vi "Subvi pixelclock start stop.vi"(0 "Nframes":u8, 1 "Nlines per frame no skips":u16, 2 "Nlines per frame plus skips":u16, 3 "Nlines all":u16, 7 "Lineclock/Pixelclock":T1, 12 "Master trigger":bool, 13 "Linegate timeout":u16) -> (4 "Gated pixelclock change":bool, 6 "Preframegate":bool, 8 "Preframeclock":bool, 10 "Preframe counter":u8, 15 "Frameclock":bool)   [LabVIEW 2017]
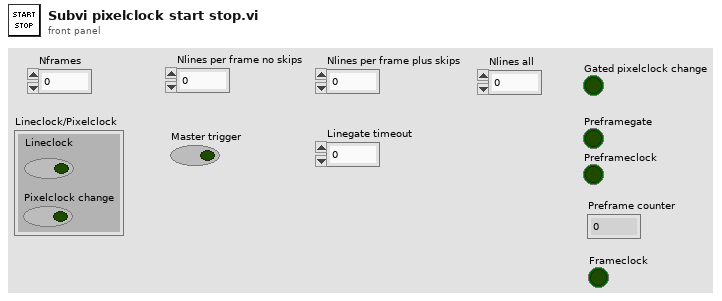
[diagram p1: front panel]
types:
  T1 = cluster{"Pixelclock change":bool, "Lineclock":bool}
  T2 = cluster{cluster{u16, "t":u8}, cluster{bool, u16, u8, bool}, cluster{bool, u16, u8, bool}}
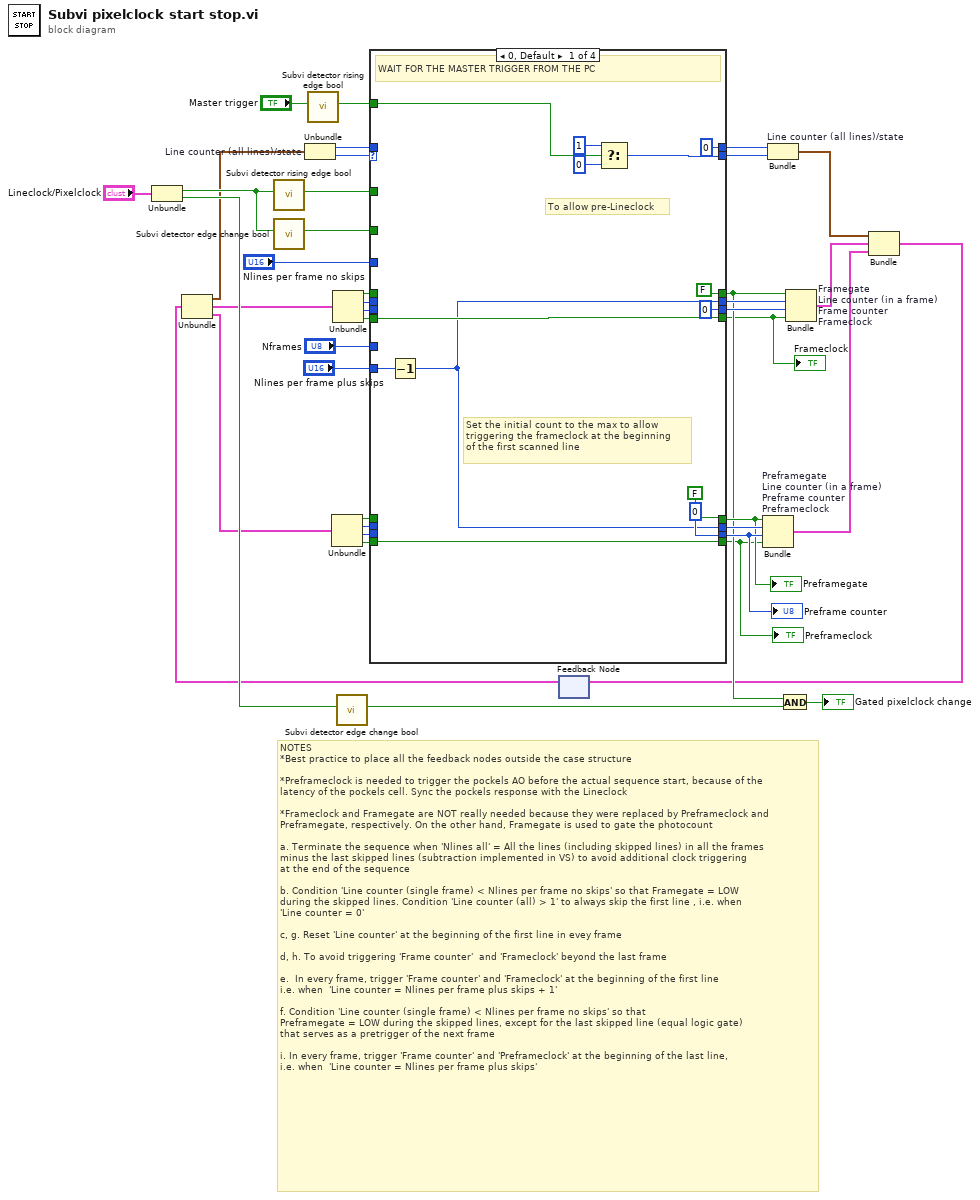
[diagram p0: block diagram]
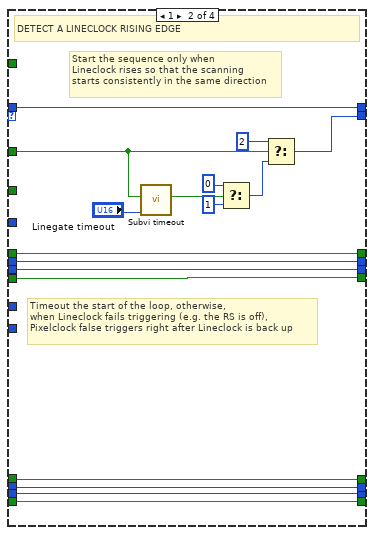
[diagram p2: hidden frame]
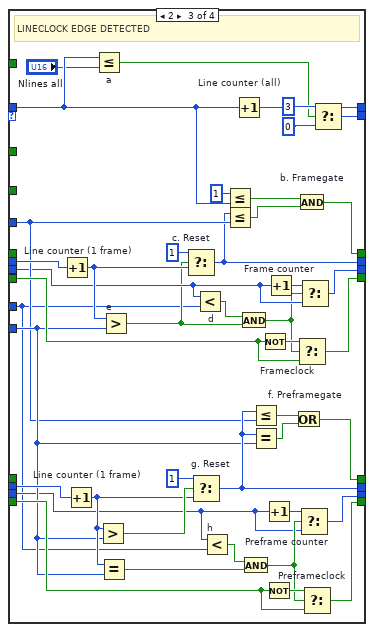
[diagram p3: hidden frame]
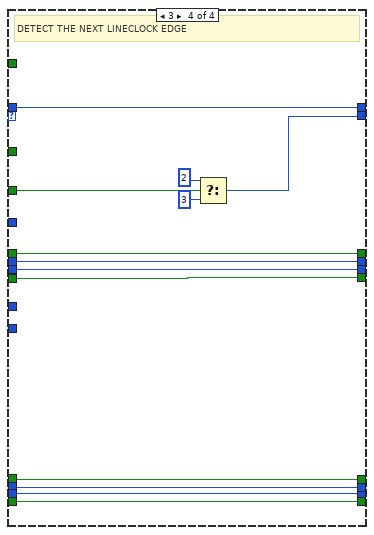
[diagram p4: hidden frame]
diagram:
  # "NOTES\n*Best practice to place all the feedback nodes outside the case structure \n\n*Preframeclock is needed to trigger the pockels AO before the actual sequence start, because of the\nlatency of the pockels cell. Sync the pockels response with the Lineclock\n\n*Frameclock and Framegate are NOT really needed because they were replaced by Preframeclock and \nPreframegate, respectively. On the other hand, Framegate is used to gate the photocount\n\na. Terminate the sequence when 'Nlines all' = All the lines (including skipped lines) in all the frames\nminus the last skipped lines (subtraction implemented in VS) to avoid additional clock triggering\nat the end of the sequence\n\nb. Condition 'Line counter (single frame) < Nlines per frame no skips' so that Framegate = LOW\nduring the skipped lines. Condition 'Line counter (all) > 1' to always skip the first line , i.e. when\n'Line counter = 0'\n\nc, g. Reset 'Line counter' at the beginning of the first line in evey frame\n\nd, h. To avoid triggering 'Frame counter'  and 'Frameclock' beyond the last frame\n\ne.  In every frame, trigger 'Frame counter' and 'Frameclock' at the beginning of the first line\ni.e. when  'Line counter = Nlines per frame plus skips + 1'\n\nf. Condition 'Line counter (single frame) < Nlines per frame no skips' so that\nPreframegate = LOW during the skipped lines, except for the last skipped line (equal logic gate)\nthat serves as a pretrigger of the next frame\n\ni. In every frame, trigger 'Frame counter' and 'Preframeclock' at the beginning of the last line,\ni.e. when  'Line counter = Nlines per frame plus skips'"
  n1 = Unbundle("Lineclock/Pixelclock") -> ("Pixelclock change"=w30:bool, "Lineclock"=w29:bool)
  n2 = call "Subvi detector rising edge bool.vi"("Input"=w30) -> ("Output"=w1:bool)  [unwired: 10 in]
  n3 = call "Subvi detector edge change bool.vi"("Input"=w30) -> ("Output"=w31:bool)  [unwired: 8 in]
  n4 = call "Subvi detector rising edge bool.vi"("Input"="Master trigger") -> ("Output"=w2:bool)  [unwired: 10 in]
  n5 = call "Subvi detector edge change bool.vi"("Input"=w29) -> ("Output"=w28:bool)  [unwired: 8 in]
  n6 = feedback #1() -> (w9:T2)  [unwired: 1 in]
  n7 = Unbundle(w9) -> (w6:cluster{u16, "t":u8}, w7:cluster{bool, u16, u8, bool}, w8:cluster{bool, u16, u8, bool})
  n8 = Unbundle "Line counter (all lines)/state"(w6) -> (w38:u16, "t"=w35:u8)
  n9 = Unbundle(w8) -> (w18:bool, w21:u16, w20:u8, w19:bool)
  n10 = Unbundle(w7) -> (w24:bool, w26:u16, w25:u8, w27:bool)
  n11 = case shown="0, Default" w35 {
    tunnel: w38 -> [_ w64 w82 w127]
    tunnel: [u16 0 w64 w99 w127] -> w39
    tunnel: [w52 w69 w107 w125] -> w37
    tunnel: [w51 w68 w112 w123] -> w4
    tunnel: w27 -> [w51 w68 w106 w123]
    tunnel: [w42 w62 w83 w121] -> w34
    tunnel: w26 -> [_ w62 w92 w121]
    tunnel: [FALSE w58 w85 w116] -> w15
    tunnel: [u8 0 w63 w110 w122] -> w33
    tunnel: w25 -> [_ w63 w75 w122]
    tunnel: w1 -> [_ w56 _ _]
    tunnel: w31 -> [_ _ _ w120]
    tunnel: w2 -> [w41 _ _ _]
    tunnel: "Nlines per frame plus skips" -> [w43 _ w89 _]
    tunnel: [w42 w61 w96 w119] -> w22
    tunnel: w21 -> [_ w61 w97 w119]
    tunnel: [u8 0 w60 w103 w118] -> w17
    tunnel: w20 -> [_ w60 w76 w118]
    tunnel: [w45 w59 w101 w117] -> w3
    tunnel: w19 -> [w45 w59 w100 w117]
    tunnel: w24 -> [_ w58 _ w116]
    tunnel: "Nframes" -> [_ _ w71 _]
    tunnel: [FALSE w57 w94 w115] -> w16
    tunnel: w18 -> [_ w57 _ w115]
    tunnel: "Nlines per frame no skips" -> [_ _ w88 _]
    frame 0, Default {
      # "To allow pre-Lineclock"
      # "Set the initial count to the max to allow\ntriggering the frameclock at the beginning\nof the first scanned line"
      # "WAIT FOR THE MASTER TRIGGER FROM THE PC"
      n12 = Decrement(x=w43) -> (x-1=w42:u16)
      n13 = Select(t=u8 1, s=w41, f=u8 0) -> (s? t:f=w52:u8)
    }
    frame 1 {
      # "Start the sequence only when\nLineclock rises so that the scanning\nstarts consistently in the same direction"
      # "Timeout the start of the loop, otherwise,\nwhen Lineclock fails triggering (e.g. the RS is off), \nPixelclock false triggers right after Lineclock is back up"
      # "DETECT A LINECLOCK RISING EDGE"
      n14 = call "Subvi timeout.vi"("Timeout_tick"="Linegate timeout", "Input"=w56) -> ("Timeout"=w55:bool)  [unwired: 9 in]
      n15 = Select(t=u8 0 ("f"), s=w55, f=u8 1) -> (s? t:f=w65:u8)
      n16 = Select(t=u8 2, s=w56, f=w65) -> (s? t:f=w69:u8)
    }
    frame 2 {
      # "LINECLOCK EDGE DETECTED"
      n17 = Increment "Line counter (1 frame)"(x=w92) -> (x+1=w90:u16)
      n18 = Increment "Line counter (1 frame)"(x=w97) -> (x+1=w91:u16)
      n19 = Less Or Equal? "a"(x=w82, y="Nlines all") -> (x <= y?=w80:bool)
      n20 = Greater?(x=w91, y=w89) -> (0:w98:bool)
      n21 = Equal?(x=w91, y=w89) -> (x = y?=w78:bool)
      n22 = Greater? "e"(x=w90, y=w89) -> (0:w72:bool)
      n23 = Select "c. Reset"(t=u16 1, s=w72, f=w90) -> (s? t:f=w83:u16)
      n24 = Select "g. Reset"(t=u16 1, s=w98, f=w91) -> (s? t:f=w96:u16)
      n25 = Less? "d"(x=w75, y=w71) -> (x < y?=w74:bool)
      n26 = Less? "h"(x=w76, y=w71) -> (x < y?=w79:bool)
      n27 = Less Or Equal?(x=u16 1, y=w82) -> (x <= y?=w86:bool)
      n28 = Less Or Equal?(x=w83, y=w88) -> (x <= y?=w87:bool)
      n29 = Increment "Line counter (all)"(x=w82) -> (x+1=w99:u16)
      n30 = And(x=w74, y=w72) -> (x .and. y?=w73:bool)
      n31 = And(x=w79, y=w78) -> (x .and. y?=w77:bool)
      n32 = Less Or Equal?(x=w96, y=w88) -> (x <= y?=w95:bool)
      n33 = Equal?(x=w96, y=w89) -> (x = y?=w93:bool)
      n34 = Not(x=w106) -> (.not. x?=w114:bool)
      n35 = Increment(x=w76) -> (x+1=w104:u8)
      n36 = Not(x=w100) -> (.not. x?=w102:bool)
      n37 = Increment(x=w75) -> (x+1=w111:u8)
      n38 = Or "f. Preframegate"(x=w95, y=w93) -> (x .or. y?=w94:bool)
      n39 = And "b. Framegate"(x=w86, y=w87) -> (x .and. y?=w85:bool)
      n40 = Select "Frameclock"(t=w114, s=w73, f=w106) -> (s? t:f=w112:bool)
      n41 = Select "Preframe counter"(t=w104, s=w77, f=w76) -> (s? t:f=w103:u8)
      n42 = Select "Frame counter"(t=w111, s=w73, f=w75) -> (s? t:f=w110:u8)
      n43 = Select "Preframeclock"(t=w102, s=w77, f=w100) -> (s? t:f=w101:bool)
      n44 = Select(t=u8 3, s=w80, f=u8 0) -> (s? t:f=w107:u8)
    }
    frame 3 {
      # "DETECT THE NEXT LINECLOCK EDGE"
      n45 = Select(t=u8 2, s=w120, f=u8 3) -> (s? t:f=w125:u8)
    }
  }
  "Preframegate" <- w16
  "Preframeclock" <- w3
  "Preframe counter" <- w17
  "Frameclock" <- w4
  n46 = Bundle "Preframegate\nLine counter (in a frame)\nPreframe counter\nPreframeclock"(w16, w22, w17, w3) -> (w11:cluster{bool, u16, u8, bool})  [unwired: 1 in]
  n47 = Bundle "Line counter (all lines)/state"(w39, "t"=w37) -> (w12:cluster{u16, "t":u8})  [unwired: 1 in]
  n48 = And(x=w15, y=w28) -> (x .and. y?=→"Gated pixelclock change":bool)
  n49 = Bundle "Framegate\nLine counter (in a frame)\nFrame counter\nFrameclock"(w15, w34, w33, w4) -> (w5:cluster{bool, u16, u8, bool})  [unwired: 1 in]
  n50 = Bundle(w12, w5, w11) -> (w10:T2)  [unwired: 1 in]
  n51 = feedback-in #1(w10) -> ()
